vi "simulatedSignalSubVI.vi"(11 "Channel":T1) -> (3 "Data":dbl)   [LabVIEW 2019]
panel:
  in  "Previous data":dbl
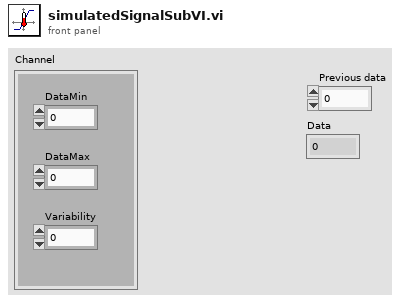
[diagram p1: front panel]
types:
  T1 = cluster{"DataMin":dbl, "DataMax":dbl, "Variability":dbl}
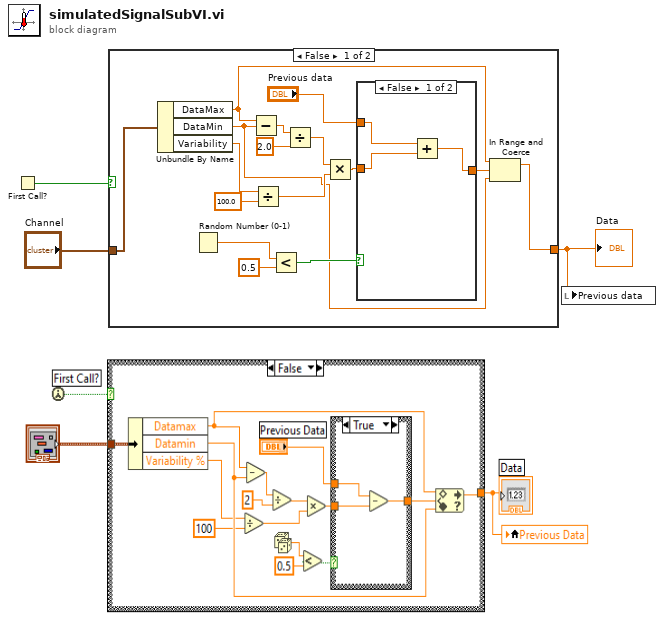
[diagram p0: block diagram]
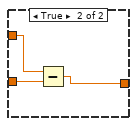
[diagram p2: hidden frame]
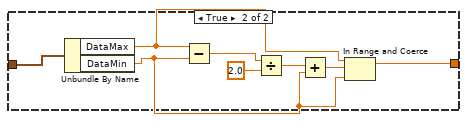
[diagram p3: hidden frame]
diagram:
  n1 = First Call?() -> (First Call?: T/F=w2:bool)
  n2 = case shown="False" w2 {
    tunnel: "Channel" -> [w19 w33]
    tunnel: [w8 w26] -> w1
    frame False {
      n3 = Unbundle By Name(w19) -> ("DataMax"=w6:dbl, "DataMin"=w5:dbl, "Variability"=w11:dbl)
      n4 = Random Number (0-1)() -> (number: 0 to 1=w16:dbl)
      n5 = Subtract(x=w6, y=w5) -> (x-y=w14:dbl)
      n6 = Divide(x=w11, y=100.0) -> (x/y=w9:dbl)
      n7 = Less?(x=w16, y=0.5) -> (x < y?=w18:bool)
      n8 = Divide(x=w14, y=2.0) -> (x/y=w13:dbl)
      n9 = Multiply(x=w13, y=w9) -> (x*y=w12:dbl)
      n10 = case shown="False" w18 {
        tunnel: "Previous data" -> [w22 w25]
        tunnel: w12 -> [w21 w24]
        tunnel: [w20 w23] -> w7
        frame False {
          n11 = Add(x=w22, y=w21) -> (x+y=w20:dbl)
        }
        frame True {
          n12 = Subtract(x=w25, y=w24) -> (x-y=w23:dbl)
        }
      }
      n13 = In Range and Coerce(upper limit=w6, x=w7, lower limit=w5) -> (coerced(x)=w8:dbl)  [unwired: 1 out]
    }
    frame True {
      n14 = Unbundle By Name(w33) -> ("DataMax"=w28:dbl, "DataMin"=w27:dbl)
      n15 = Subtract(x=w28, y=w27) -> (x-y=w31:dbl)
      n16 = Divide(x=w31, y=2.0) -> (x/y=w29:dbl)
      n17 = Add(x=w29, y=w27) -> (x+y=w30:dbl)
      n18 = In Range and Coerce(upper limit=w28, x=w30, lower limit=w27) -> (coerced(x)=w26:dbl)  [unwired: 1 out]
    }
  }
  "Data" <- w1
  n19 = local write "Previous data"(w1) -> ()
